vi "DOE Calculate Rinse Gallons.vi"(6 "Hot Water Total During Wash (Gal)":dbl, 8 "Error In":errorcluster, 9 "Cold Water Total During Wash (Gal)":dbl, 10 "Hot Water Total (Gal)":dbl, 11 "Cold Water Total (Gal)":dbl) -> (0 "Error Out":errorcluster, 2 "Rinse_HW":dbl, 3 "Rinse_CW":dbl)   [LabVIEW 2019]
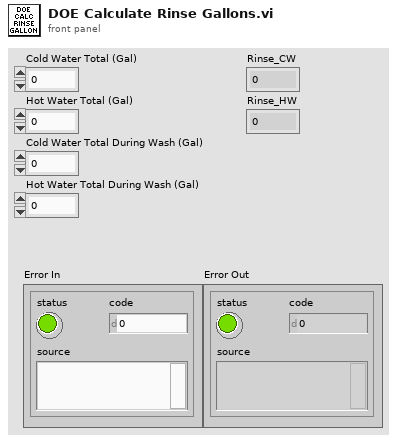
[diagram p1: front panel]
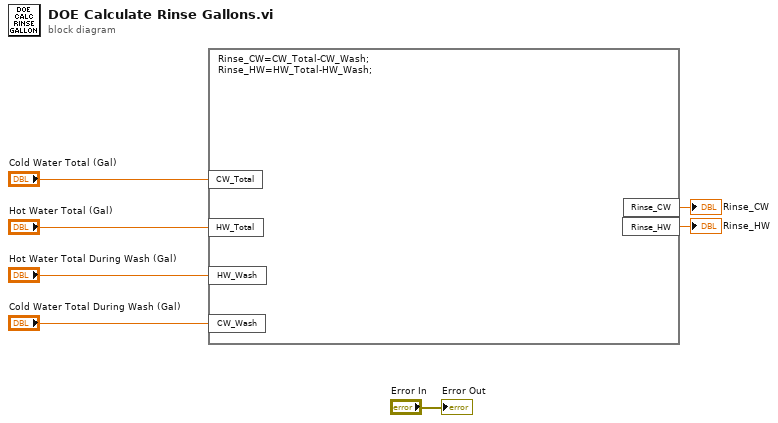
[diagram p0: block diagram]
diagram:
  n1 = formula code="Rinse_CW=CW_Total-CW_Wash;\nRinse_HW=HW_Total-HW_Wash;"("HW_Total"="Hot Water Total (Gal)", "CW_Total"="Cold Water Total (Gal)", "HW_Wash"="Hot Water Total During Wash (Gal)", "CW_Wash"="Cold Water Total During Wash (Gal)") -> ("Rinse_CW"=→"Rinse_CW":dbl, "Rinse_HW"=→"Rinse_HW":dbl)
  "Error Out" <- "Error In"
